vi "N3.vi"() -> ()   [LabVIEW 2020]
uses:
  <vilib>/numeric/Random Number (Range) I64.vi
  <vilib>/numeric/sub_Random U32.vi
panel:
  out "Waveform Graph":i64[][](graph)
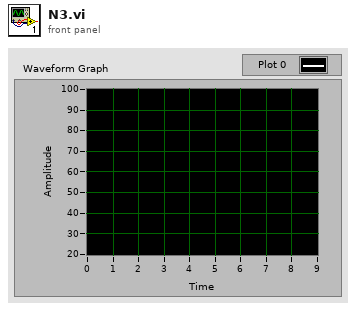
[diagram p1: front panel]
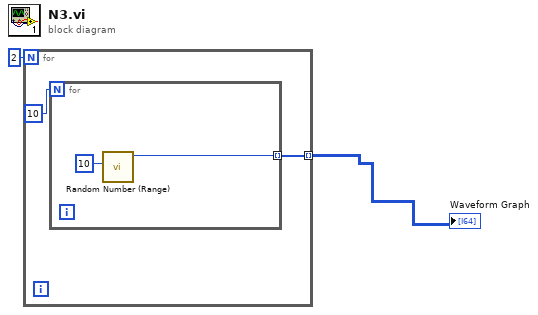
[diagram p0: block diagram]
diagram:
  n1 = for {
    N: 2 -> [_]
    tunnel: [w3] -> w1 mode=indexing
    n2 = for {
      N: 10 -> [_]
      tunnel: [w6] -> w3 mode=indexing
      n3 = call-poly <vilib>:"Random Number (Range).vi"("lower bound (-100)"=i64 10) -> ("number"=w6:i64)  [unwired: 10 in]
    }
  }
  "Waveform Graph" <- w1
